vi "IV Curve.vi"() -> ()   [LabVIEW 2018]
uses:
  <vilib>/Analysis/baseanly.llb/Mean (DBL).vi
  <vilib>/express/express shared/transition.llb/Dynamic To Waveform Array.vi
  <vilib>/express/express signal manip/GetorSetDDTAttributes/Set DDT Attributes/SetT0.vi
  <vilib>/express/express shared/transition.llb/Waveform Array To Dynamic.vi
  <vilib>/express/express signal manip/GetorSetDDTAttributes/Set DDT Attributes/Set DDT Properties.xnode
  <instrlib>/XP Power PLS600/XP Power PLS600.lvlib
  <vilib>/Analysis/NI_AALBase.lvlib
panel:
  in  "stop":bool
  out "Voltage level":dbl format="%#_13g"
  out "Current level":dbl format="%#_13g"
  in  "Filename":path=path "C:/Users/mtree/Desktop/testing.xls"
  out "Current\n Voltage for FP 2":dbl=6.999999999999991 format="%#_13g"
  in  "Changing Voltage":dbl format="%#_13g"
  in  "Voltage Max":dbl format="%#_13g"
  in  "Set Current Limit for FP":dbl=1.0 format="%#_13g"
  in  "Start Voltage for FP":dbl format="%#_13g"
  in  "VISA resource name":refnum<visa-resource-name>
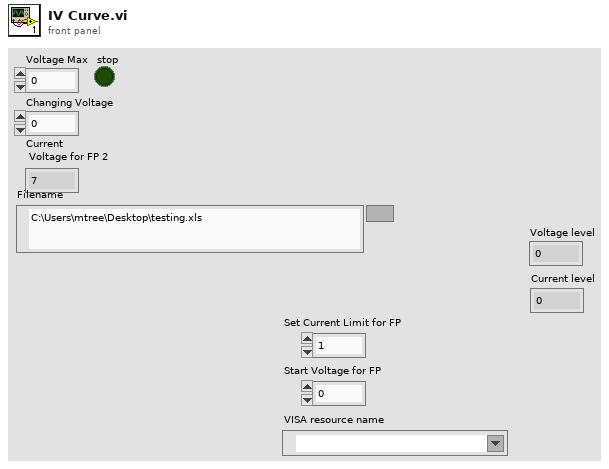
[diagram p1: front panel]
types:
  T1 = cluster{"Baud Rate":u32, "Parity":u16, "Data Bits":u16, "Stop Bits":u16, "Flow Control":u16}
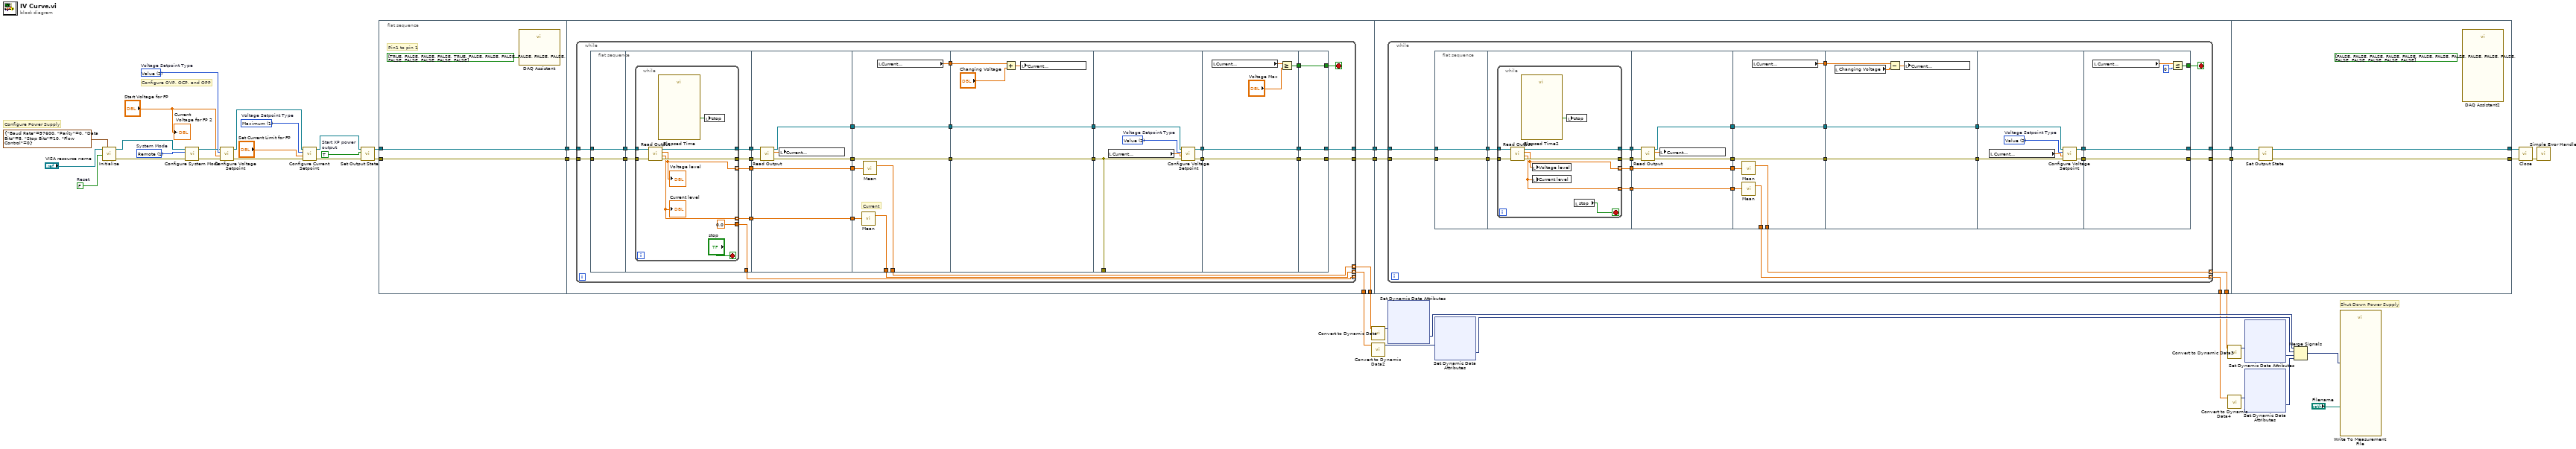
[diagram p0: block diagram]
diagram:
  w29 = 1 items=["Minimum", "Maximum", "Value"]  # Voltage Setpoint Type
  w39 = TRUE  # Start XP power output
  w37 = 2 items=["Minimum", "Maximum", "Value"]  # Voltage Setpoint Type
  w38 = 1 items=["Local", "Remote", "Remote with Lock", "Voltage", "Current", "Dual"]  # System Mode
  w35 = FALSE  # Reset
  # "Shut Down Power Supply"
  # "Configure Power Supply"
  # "Configure OVP, OCP, and OPP"
  n1 = call <instrlib>:"Initialize.vi"("Serial Configuration"=T1 {"Baud Rate"=57600, "Parity"=0, "Data Bits"=8, "Stop Bits"=10, "Flow Control"=0}, "Reset (True)"=w35, "VISA resource name"="VISA resource name") -> ("error out"=w42:errorcluster, "VISA resource name out"=w41:refnum<visa-resource-name>)  [unwired: 7 in]
  n2 = call <instrlib>:"Configure System Mode.vi"("error in (no error)"=w42, "System Mode (0: Local)"=w38, "VISA resource name"=w41) -> ("error out"=w27:errorcluster, "VISA resource name out"=w28:refnum<visa-resource-name>)  [unwired: 7 in]
  n3 = call <instrlib>:"Configure Voltage Setpoint.vi"("error in (no error)"=w27, "Voltage Setpoint (0 volts)"="Start Voltage for FP", "Voltage Setpoint Type (0: Minimum)"=w37, "VISA resource name"=w28) -> ("error out"=w31:errorcluster, "VISA resource name out"=w34:refnum<visa-resource-name>)  [unwired: 6 in]
  n4 = call <instrlib>:"Configure Current Setpoint.vi"("error in (no error)"=w31, "Current Setpoint (0 amperes)"="Set Current Limit for FP", "Current Setpoint Type (0: Minimum)"=w29, "VISA resource name"=w34) -> ("error out"=w32:errorcluster, "VISA resource name out"=w33:refnum<visa-resource-name>)  [unwired: 6 in]
  n5 = call <instrlib>:"Set Output State.vi"("error in (no error)"=w32, "Output State (F: Disable)"=w39, "VISA resource name"=w33) -> ("error out"=w22:errorcluster, "VISA resource name out"=w24:refnum<visa-resource-name>)  [unwired: 7 in]
  n6 = flat-sequence {
    tunnel: [w45] -> w25
    tunnel: w24 -> [w45]
    tunnel: [w44] -> w23
    tunnel: w22 -> [w44]
    tunnel: [w48] -> w12
    tunnel: w25 -> [w51]
    tunnel: [w50] -> w10
    tunnel: w23 -> [w49]
    tunnel: [w47] -> w14
    tunnel: [w46] -> w13
    tunnel: w12 -> [w135]
    tunnel: [w136] -> w11
    tunnel: w10 -> [w133]
    tunnel: [w134] -> w9
    tunnel: [w132] -> w2
    tunnel: [w131] -> w1
    tunnel: w11 -> [w209]
    tunnel: w9 -> [w210]
    tunnel: [w208] -> w8
    tunnel: [w207] -> w7
    frame #0 {
      # "Pin1 to pin 1"
      n7 = call "DAQ Assistant"("data"=bool[] [TRUE, FALSE, FALSE, FALSE, TRUE, FALSE, FALSE, FALSE, FALSE, FALSE, FALSE, FALSE, FALSE, FALSE, FALSE, FALSE]) -> ()  [unwired: 17 in, 2 out]
    }
    frame #1 {
      n8 = while {
        tunnel: w51 -> [w76]
        tunnel: [w75] -> w50
        tunnel: w49 -> [w67]
        tunnel: [w79] -> w48
        tunnel: [w72] -> w47 mode=indexing
        tunnel: [w64] -> w46 mode=indexing
        tunnel: [w55] -> _ mode=indexing
        stop <- w69 stop-if-true
        n9 = flat-sequence {
          tunnel: w76 -> [w81]
          tunnel: [w81] -> w74
          tunnel: [w80] -> w68
          tunnel: w67 -> [w80]
          tunnel: [w85] -> w63
          tunnel: w74 -> [w86]
          tunnel: w68 -> [w88]
          tunnel: [w87] -> w61
          tunnel: [w84] -> w59
          tunnel: [w83] -> w57
          tunnel: [w82] -> w55
          tunnel: w63 -> [w100]
          tunnel: [w99] -> w62
          tunnel: w61 -> [w102]
          tunnel: [w101] -> w60
          tunnel: w59 -> [w104]
          tunnel: [w104] -> w58
          tunnel: w57 -> [w103]
          tunnel: [w103] -> w56
          tunnel: [w111] -> w77
          tunnel: w62 -> [w111]
          tunnel: [w110] -> w73
          tunnel: [w107] -> w72
          tunnel: [w109] -> w65
          tunnel: w60 -> [w109]
          tunnel: w58 -> [w108]
          tunnel: w56 -> [w106]
          tunnel: [w105] -> w64
          tunnel: [w116] -> w78
          tunnel: w77 -> [w116]
          tunnel: w73 -> [w113]
          tunnel: [w112] -> w66
          tunnel: w65 -> [w112]
          tunnel: w78 -> [w121]
          tunnel: [w117] -> _
          tunnel: [w120] -> w71
          tunnel: [w119] -> w70
          tunnel: w66 -> [w117]
          tunnel: w71 -> [w127]
          tunnel: w70 -> [w126]
          tunnel: [w127] -> w54
          tunnel: [w126] -> w53
          tunnel: [w123] -> w52
          tunnel: [w128] -> w69
          tunnel: [w129] -> w75
          tunnel: [w130] -> w79
          tunnel: w54 -> [w130]
          tunnel: w53 -> [w129]
          tunnel: w52 -> [w128]
          frame #0 {
          }
          frame #1 {
            n10 = while {
              tunnel: w88 -> [w97]
              tunnel: [w96] -> w87
              tunnel: w86 -> [w95]
              tunnel: [w94] -> w85
              tunnel: [w93] -> w84 mode=indexing
              tunnel: [w91] -> w83 mode=indexing
              tunnel: [0.0] -> w82
              stop <- "stop" stop-if-true
              n11 = call <instrlib>:"Read Output.vi"("error in (no error)"=w97, "VISA resource name"=w95) -> ("error out"=w96:errorcluster, "Actual Current Level (amperes)"=w93:dbl, "Actual Voltage Level (volts)"=w91:dbl, "VISA resource name out"=w94:refnum<visa-resource-name>)  [unwired: 6 in]
              "Current level" <- w93
              "Voltage level" <- w91
              n12 = call "Elapsed Time"() -> ("Time has Elapsed"=w90:bool)  [unwired: 12 in, 7 out]
              n13 = local write "stop"(w90) -> ()
            }
          }
          frame #2 {
            n14 = call <instrlib>:"Read Output.vi"("error in (no error)"=w102, "VISA resource name"=w100) -> ("error out"=w101:errorcluster, "Actual Voltage Level (volts)"=w98:dbl, "VISA resource name out"=w99:refnum<visa-resource-name>)  [unwired: 6 in, 1 out]
            n15 = local write "Current\n Voltage for FP 2"(w98) -> ()
          }
          frame #3 {
            # "Current"
            n16 = call-poly <vilib>:"Mean.vi"("X"=w108) -> ("mean"=w107:dbl)  [unwired: 1 out]
            n17 = call-poly <vilib>:"Mean.vi"("X"=w106) -> ("mean"=w105:dbl)  [unwired: 1 out]
            n18 = local read "Current\n Voltage for FP 2"() -> (w110:dbl)
          }
          frame #4 {
            n19 = Add(x=w113, y="Changing Voltage") -> (x+y=w114:dbl)
            n20 = local write "Current\n Voltage for FP 2"(w114) -> ()
          }
          frame #5 {
            w118 = 2 items=["Minimum", "Maximum", "Value"]  # Voltage Setpoint Type
            n21 = local read "Current\n Voltage for FP 2"() -> (w122:dbl)
            n22 = call <instrlib>:"Configure Voltage Setpoint.vi"("error in (no error)"=w117, "Voltage Setpoint (0 volts)"=w122, "Voltage Setpoint Type (0: Minimum)"=w118, "VISA resource name"=w121) -> ("error out"=w119:errorcluster, "VISA resource name out"=w120:refnum<visa-resource-name>)  [unwired: 6 in]
          }
          frame #6 {
            n23 = local read "Current\n Voltage for FP 2"() -> (w124:dbl)
            n24 = Greater Or Equal?(x=w124, y="Voltage Max") -> (x >= y?=w123:bool)
          }
          frame #7 {
          }
        }
      }
    }
    frame #2 {
      n25 = while {
        tunnel: [w160] -> w136
        tunnel: w135 -> [w153]
        tunnel: [w152] -> w134
        tunnel: w133 -> [w145]
        tunnel: [w140] -> w132 mode=indexing
        tunnel: [w139] -> w131 mode=indexing
        stop <- w137 stop-if-true
        n26 = flat-sequence {
          tunnel: [w162] -> w154
          tunnel: w153 -> [w162]
          tunnel: [w161] -> w146
          tunnel: w145 -> [w161]
          tunnel: [w166] -> w155
          tunnel: w154 -> [w168]
          tunnel: [w165] -> w147
          tunnel: w146 -> [w167]
          tunnel: [w164] -> w143
          tunnel: [w163] -> w141
          tunnel: [w181] -> w156
          tunnel: w155 -> [w183]
          tunnel: [w180] -> w148
          tunnel: w147 -> [w182]
          tunnel: [w178] -> w144
          tunnel: w143 -> [w178]
          tunnel: [w177] -> w142
          tunnel: w141 -> [w177]
          tunnel: [w190] -> w157
          tunnel: w156 -> [w190]
          tunnel: [w189] -> w149
          tunnel: w148 -> [w189]
          tunnel: w144 -> [w188]
          tunnel: w142 -> [w187]
          tunnel: [w186] -> w140
          tunnel: [w185] -> w139
          tunnel: [w184] -> w138
          tunnel: [w195] -> w158
          tunnel: w157 -> [w195]
          tunnel: [w194] -> w150
          tunnel: w149 -> [w194]
          tunnel: w138 -> [w192]
          tunnel: [w196] -> w159
          tunnel: w158 -> [w199]
          tunnel: [w197] -> w151
          tunnel: w150 -> [w198]
          tunnel: [w206] -> w160
          tunnel: w159 -> [w206]
          tunnel: [w205] -> w152
          tunnel: w151 -> [w205]
          tunnel: [w202] -> w137
          frame #0 {
          }
          frame #1 {
            n27 = while {
              tunnel: w168 -> [w175]
              tunnel: w167 -> [w174]
              tunnel: [w173] -> w166
              tunnel: [w172] -> w165
              tunnel: [w171] -> w164 mode=indexing
              tunnel: [w170] -> w163 mode=indexing
              stop <- w169 stop-if-true
              n28 = call <instrlib>:"Read Output.vi"("error in (no error)"=w174, "VISA resource name"=w175) -> ("error out"=w172:errorcluster, "Actual Current Level (amperes)"=w170:dbl, "Actual Voltage Level (volts)"=w171:dbl, "VISA resource name out"=w173:refnum<visa-resource-name>)  [unwired: 6 in]
              n29 = call "Elapsed Time2"() -> ("Time has Elapsed"=w176:bool)  [unwired: 12 in, 7 out]
              n30 = local write "Voltage level"(w171) -> ()
              n31 = local write "Current level"(w170) -> ()
              n32 = local write "stop"(w176) -> ()
              n33 = local read "stop"() -> (w169:bool)
            }
          }
          frame #2 {
            n34 = call <instrlib>:"Read Output.vi"("error in (no error)"=w182, "VISA resource name"=w183) -> ("error out"=w180:errorcluster, "Actual Voltage Level (volts)"=w179:dbl, "VISA resource name out"=w181:refnum<visa-resource-name>)  [unwired: 6 in, 1 out]
            n35 = local write "Current\n Voltage for FP 2"(w179) -> ()
          }
          frame #3 {
            n36 = call-poly <vilib>:"Mean.vi"("X"=w188) -> ("mean"=w186:dbl)  [unwired: 1 out]
            n37 = call-poly <vilib>:"Mean.vi"("X"=w187) -> ("mean"=w185:dbl)  [unwired: 1 out]
            n38 = local read "Current\n Voltage for FP 2"() -> (w184:dbl)
          }
          frame #4 {
            n39 = local read "Changing Voltage"() -> (w191:dbl)
            n40 = Subtract(x=w192, y=w191) -> (x-y=w193:dbl)
            n41 = local write "Current\n Voltage for FP 2"(w193) -> ()
          }
          frame #5 {
            w200 = 2 items=["Minimum", "Maximum", "Value"]  # Voltage Setpoint Type
            n42 = local read "Current\n Voltage for FP 2"() -> (w201:dbl)
            n43 = call <instrlib>:"Configure Voltage Setpoint.vi"("error in (no error)"=w198, "Voltage Setpoint (0 volts)"=w201, "Voltage Setpoint Type (0: Minimum)"=w200, "VISA resource name"=w199) -> ("error out"=w197:errorcluster, "VISA resource name out"=w196:refnum<visa-resource-name>)  [unwired: 6 in]
          }
          frame #6 {
            n44 = local read "Current\n Voltage for FP 2"() -> (w203:dbl)
            n45 = Less Or Equal?(x=w203, y=0) -> (x <= y?=w202:bool)
          }
        }
      }
    }
    frame #3 {
      n46 = call <instrlib>:"Set Output State.vi"("error in (no error)"=w210, "VISA resource name"=w209) -> ("error out"=w208:errorcluster, "VISA resource name out"=w207:refnum<visa-resource-name>)  [unwired: 8 in]
      n47 = call "DAQ Assistant2"("data"=bool[] [FALSE, FALSE, FALSE, FALSE, FALSE, FALSE, FALSE, FALSE, FALSE, FALSE, FALSE, FALSE, FALSE, FALSE, FALSE, FALSE]) -> ()  [unwired: 17 in, 2 out]
    }
  }
  n48 = call "Convert to Dynamic Data"("Array"=w13) -> ("Dynamic Data Type"=w19:dynamicdata)  [unwired: 3 in]
  n49 = call "Convert to Dynamic Data2"("Array"=w14) -> ("Dynamic Data Type"=w17:dynamicdata)  [unwired: 3 in]
  n50 = xnode "Set Dynamic Data Attributes"("Signals In"=w19) -> ("Signals Out"=w18:dynamicdata)  [unwired: 3 in, 1 out]
  n51 = xnode "Set Dynamic Data Attributes"("Signals In"=w17) -> ("Signals Out"=w16:dynamicdata)  [unwired: 3 in, 1 out]
  n52 = call "Convert to Dynamic Data3"("Array"=w2) -> ("Dynamic Data Type"=w6:dynamicdata)  [unwired: 3 in]
  n53 = call "Convert to Dynamic Data4"("Array"=w1) -> ("Dynamic Data Type"=w5:dynamicdata)  [unwired: 3 in]
  n54 = xnode "Set Dynamic Data Attributes"("Signals In"=w6) -> ("Signals Out"=w4:dynamicdata)  [unwired: 3 in, 1 out]
  n55 = xnode "Set Dynamic Data Attributes"("Signals In"=w5) -> ("Signals Out"=w3:dynamicdata)  [unwired: 3 in, 1 out]
  n56 = Merge Signals(w18, w16, w4, w3) -> (w15:dynamicdata)
  n57 = call "Write To Measurement File"("Signals"=w15, "Filename"="Filename") -> ()  [unwired: 15 in, 3 out]
  n58 = call <instrlib>:"Close.vi"("error in (no error)"=w8, "VISA resource name"=w7) -> ("error out"=w26:errorcluster)  [unwired: 9 in]
  n59 = call <vilib>:"Simple Error Handler.vi"("error in (no error)"=w26) -> ()  [unwired: 4 in, 5 out]
  "Current\n Voltage for FP 2" <- "Start Voltage for FP"
